vi "Write Roles.vi"(8 "error in (no error)":errorcluster, 10 "Roles":T1, 11 "PenaltyEnemyPlayVSS in":refnum<class "PenaltyEnemyPlayVSS.lvclass">) -> (0 "error out":errorcluster, 3 "PenaltyEnemyPlayVSS out":refnum<class "PenaltyEnemyPlayVSS.lvclass">)   [LabVIEW 2020, in "PenaltyEnemyPlayVSS.lvclass"]
uses:
  PenaltyEnemyPlayVSS.lvclass
  KeeperRoleVSS_class/KeeperRoleVSS.lvclass
  HaltRole_class/HaltRole.lvclass
  PenaltyEnemyPlayVSS.lvclass/PenaltyEnemyPlayVSS.ctl
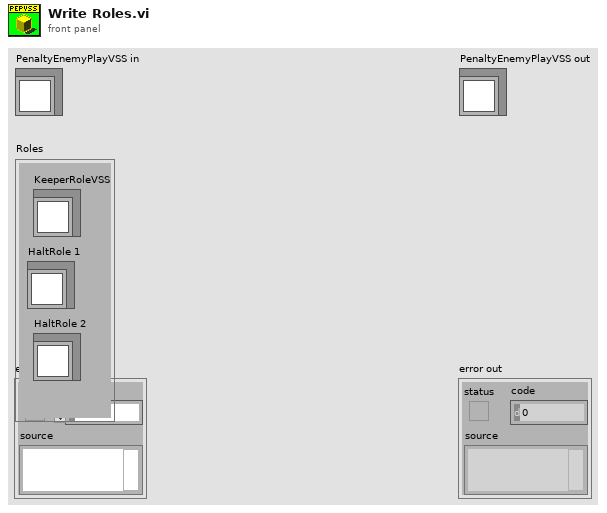
[diagram p1: front panel]
types:
  T1 = cluster{"KeeperRoleVSS":refnum<class "KeeperRoleVSS.lvclass">, "HaltRole 1":refnum<class "HaltRole.lvclass">, "HaltRole 2":refnum<class "HaltRole.lvclass">}
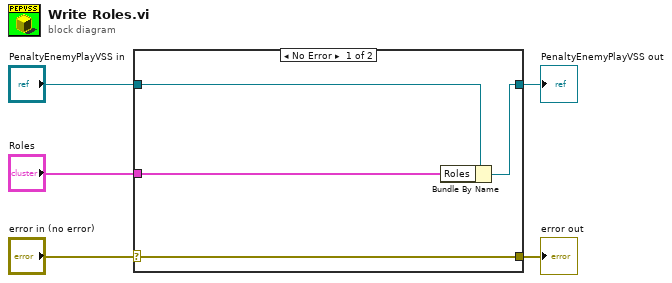
[diagram p0: block diagram]
diagram:
  n1 = case shown="No Error" "error in (no error)" {
    selector: "error in (no error)" -> [w9 w10]
    tunnel: [w9 w10] -> w4
    tunnel: [w7 w11] -> w2
    tunnel: "PenaltyEnemyPlayVSS in" -> [w8 w11]
    tunnel: "Roles" -> [w6 _]
    frame No Error {
      n2 = Bundle By Name(cluster=w8, "Roles"=w6) -> (w7:refnum<class "PenaltyEnemyPlayVSS.lvclass">)
    }
    frame Error {
    }
  }
  "error out" <- w4
  "PenaltyEnemyPlayVSS out" <- w2
